vi "TDTSyn-Get Waves (Client Side).vi"(0 "IP Address":string, 5 "Port":i32, 7 "last read":bool, 11 "error in (no error)":errorcluster, 12 "Codes":string) -> (8 "waves":dbl[][](array[numeric]), 15 "error out":errorcluster)   [LabVIEW 2020]
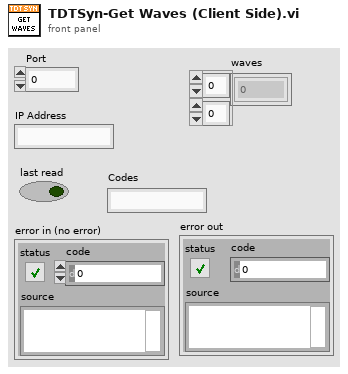
[diagram p1: front panel]
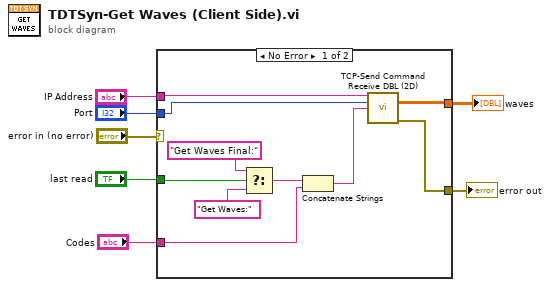
[diagram p0: block diagram]
diagram:
  n1 = case shown="No Error" "error in (no error)" {
    selector: "error in (no error)" -> [_ w18]
    tunnel: "IP Address" -> [w15 _]
    tunnel: "Port" -> [w14 _]
    tunnel: "last read" -> [w17 _]
    tunnel: [w13 w18] -> w3
    tunnel: "Codes" -> [w9 _]
    tunnel: [w8 _] -> w1
    frame No Error {
      n2 = Select(t="Get Waves Final:" ("Command"), s=w17, f="Get Waves:" ("Command")) -> (s? t:f=w11:string)
      n3 = Concatenate Strings(w11, w9) -> (w10:string)
      n4 = call "TCP-Send Command Receive DBL (2D).vi"("PXI Address"=w15, "Port"=w14, "Command"=w10) -> ("data"=w8:dbl[][], "error out"=w13:errorcluster)  [unwired: 10 in, 1 out]
    }
    frame Error {
    }
  }
  "error out" <- w3
  "waves" <- w1
